vi "Determine_Final_Trim.vi"(5 "Test_Limits":T1=[{"Test_Name"="ODFT_Trim", "Target"=1.9, "Reg_Add_0X00"=81, "Data_LSB"=4, "Data_Length"=4, "Settings"=[8, 9, 10, 11, 12, 13, 14, 15, 0, 1, 2, 3, 4, 5, 6, 7], "MSB_Reg_Add_0X00"=0, "Data_MSB"=0}, {"Test_Name"="HV_Trim", "Target"=39.0, "Reg_Add_0X00"=81, "Data_LSB"=0, "Data_Length"=4, "Settings"=[7, 6, 5, 4, 3, 2, 1, 0, 15, 14, 13, 12, 11, 10, 9, 8], "MSB_Reg_Add_0X00"=0, "Data_MSB"=0}, {"Test_Name"="Freq_Trim", "Target"=20.0, "Reg_Add_0X00"=80, "Data_LSB"=0, "Data_Length"=4, "Settings"=[0, 1, 2, 3, 4, 5, 6, 7, 8, 9, 10, 11, 12, 13, 14, 15], "MSB_Reg_Add_0X00"=0, "Data_MSB"=0}] {"MSB_Reg_Add_0X00" format="%.0x"; "Reg_Add_0X00" format="%.0x"}, 7 "Test_Name":string="ODFT_Trim", 10 "Trim_Array":u8[](array[numeric]), 11 "Meas_Array":dbl[](array[numeric])) -> (3 "Final_Trim Value":u8)   [LabVIEW 2013]
uses:
  Controls/Trim_Config_Settings_Array.ctl
  Controls/Trim_Config_Settings.ctl
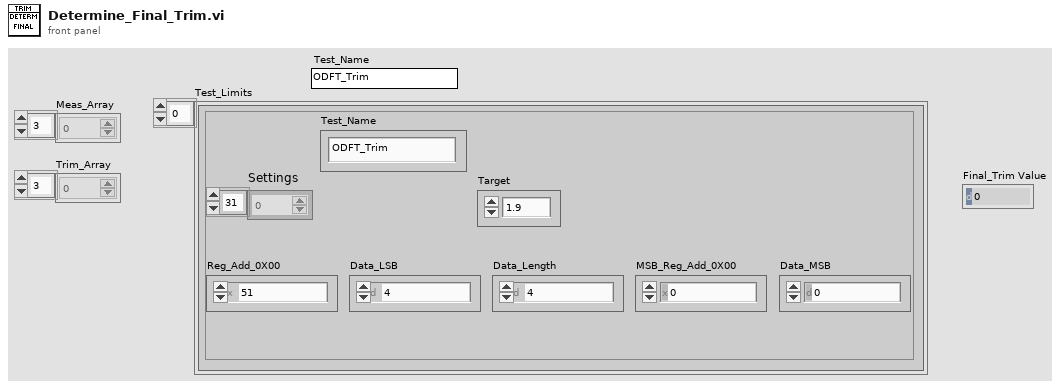
[diagram p1: front panel]
types:
  T1 = typedef "Trim_Config_Settings_Array.ctl" = T2[]
  T2 = typedef "Trim_Config_Settings.ctl" = cluster{"Test_Name":string, "Target":dbl, "Reg_Add_0X00":u8, "Data_LSB":u8, "Data_Length":u8, "Settings":u8[], "MSB_Reg_Add_0X00":u8, "Data_MSB":u8}
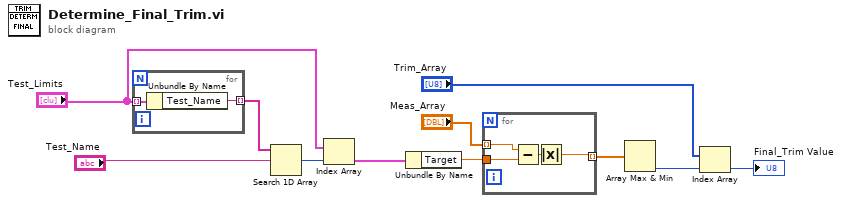
[diagram p0: block diagram]
diagram:
  n1 = for {
    tunnel: "Test_Limits" -> [w13] mode=indexing
    tunnel: [w12] -> w11 mode=indexing
    n2 = Unbundle By Name(w13) -> ("Test_Name"=w12:string)
  }
  n3 = Search 1D Array(1D array=w11, element="Test_Name") -> (index of element=w10:i32)  [unwired: 1 in]
  n4 = Index Array(array="Test_Limits", index=w10) -> (element=w9:T2)
  n5 = Unbundle By Name(w9) -> ("Target"=w4:dbl)
  n6 = for {
    tunnel: [w16] -> w6 mode=indexing
    tunnel: "Meas_Array" -> [w15] mode=indexing
    tunnel: w4 -> [w14]
    n7 = Subtract(x=w15, y=w14) -> (x-y=w17:dbl)
    n8 = Absolute Value(x=w17) -> (abs(x)=w16:dbl)
  }
  n9 = Array Max & Min(array=w6) -> (min index (indices)=w2:i32)  [unwired: 3 out]
  n10 = Index Array(array="Trim_Array", index=w2) -> (element=→"Final_Trim Value":u8)
